vi "Obtain Request Events.vi"(8 "error in":errorcluster, 10 "Create New? (F)":bool) -> (0 "error out":errorcluster, 2 "Core Request Events":T1)   [LabVIEW 2026, in "Core.lvlib"]
doc: "This VI Obtains/Creates the Requests events that will be used for other modules to communicate with the module that owns this VI. These Requests events will be accessed only via Public API methods for this module.\n\n<b>NOTE</b>: The contents of this VI are automatically generated and modified by the <b>Tools > DQMH Consortium > DQMH</b> utilities. Consider using those utilities instead of making your own modifications to this VI.\n_____\nBased on DQMH Dev Tools: Project Template 7.1.2.1547."
uses:
  Core.lvlib
  Request Events--cluster.ctl
  Stop Argument--cluster.ctl
  Show Panel Argument--cluster.ctl
  Hide Panel Argument--cluster.ctl
  Show Diagram Argument--cluster.ctl
  Get Module Execution Status Argument--cluster.ctl
  LaunchEventRecorder Argument--cluster.ctl
  Launcher/Mode.ctl
  Resubscribe to Cloneable Argument--cluster.ctl
  LaunchReplayModule Argument--cluster.ctl
panel:
  # "NOTE: The contents of this VI are automatically generated and modified by the Tools > DQMH Consortium > DQMH utilities. Consider using those utilities instead of making your own modifications to this VI."
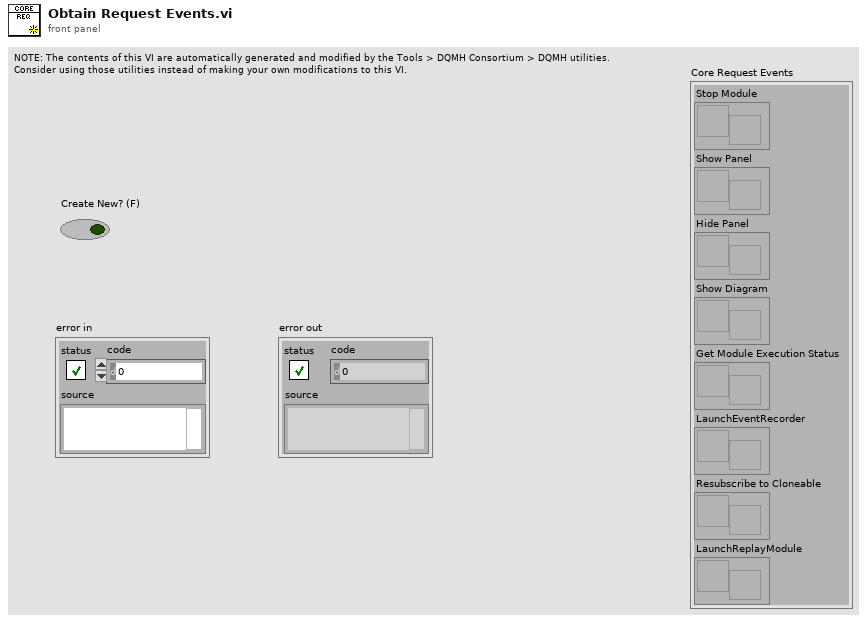
[diagram p1: front panel]
types:
  T1 = typedef "Core.lvlib/Request Events--cluster.ctl" = cluster{"Stop Module":refnum<user-event>, "Show Panel":refnum<user-event>, "Hide Panel":refnum<user-event>, "Show Diagram":refnum<user-event>, "Get Module Execution Status":refnum<user-event>, "LaunchEventRecorder":refnum<user-event>, "Resubscribe to Cloneable":refnum<user-event>, "LaunchReplayModule":refnum<user-event>}
  T2 = typedef "Core.lvlib/LaunchReplayModule Argument--cluster.ctl" = cluster{"Module ID":i32, "Run ID":string}
  T3 = typedef "Core.lvlib/Resubscribe to Cloneable Argument--cluster.ctl" = cluster{"Module ID":i32, "Boolean":bool}
  T4 = typedef "Core.lvlib/LaunchEventRecorder Argument--cluster.ctl" = cluster{"Module ID":i32, "Mode":T5}
  T5 = typedef "Mode.ctl" = enum16{"Record", "Record and Replay"}
  T6 = typedef "Core.lvlib/Get Module Execution Status Argument--cluster.ctl" = cluster{"Module ID":i32, "Running?":bool}
  T7 = typedef "Core.lvlib/Show Diagram Argument--cluster.ctl" = cluster{"Module ID":i32, "Debug?":bool}
  T8 = typedef "Core.lvlib/Show Panel Argument--cluster.ctl" = cluster{"Module ID":i32, "Show Panel?":bool}
  T9 = typedef "Core.lvlib/Hide Panel Argument--cluster.ctl" = cluster{"Module ID":i32, "Hide Panel?":bool}
  T10 = typedef "Core.lvlib/Stop Argument--cluster.ctl" = cluster{"Module ID":i32, "Origin":string, "Exit via Stop Module Req?":bool, "Wait for Module to stop?":bool}
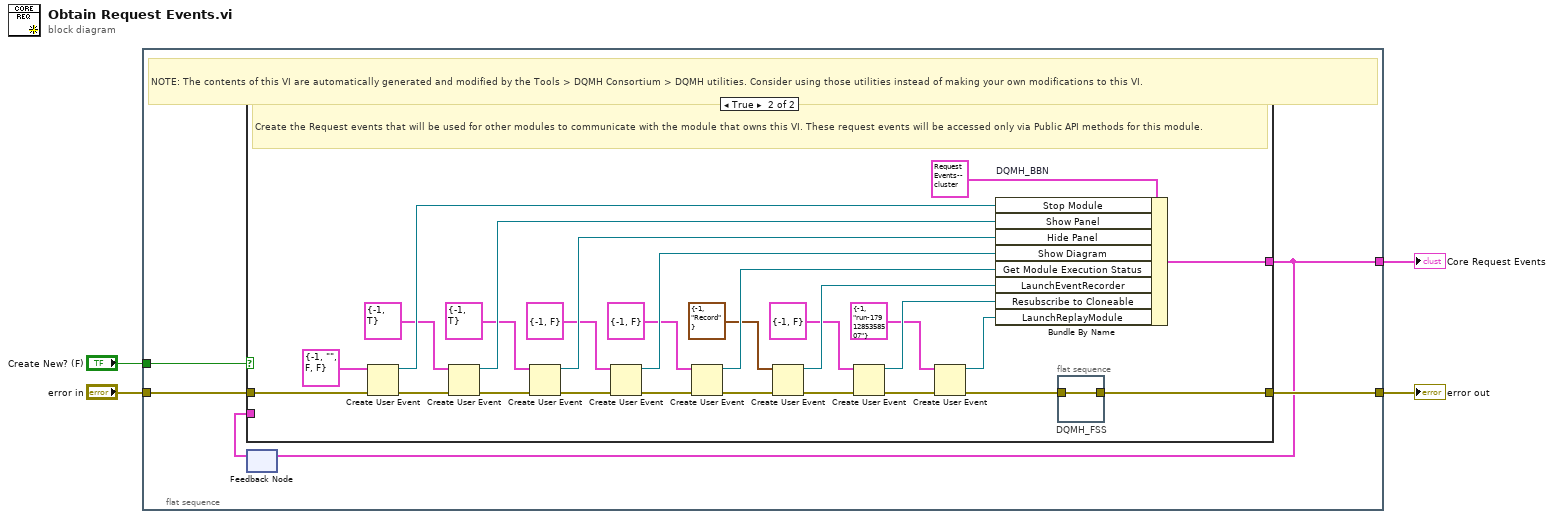
[diagram p0: block diagram]
diagram:
  n1 = flat-sequence {
    tunnel: [w9] -> w4
    tunnel: "error in" -> [w8]
    tunnel: [w6] -> w2
    tunnel: "Create New? (F)" -> [w5]
    frame #0 {
      # "NOTE: The contents of this VI are automatically generated and modified by the Tools > DQMH Consortium > DQMH utilities. Consider using those utilities instead of making your own modifications to this VI."
      n2 = feedback #1() -> (w7:T1)  [unwired: 1 in]
      n3 = case shown="True" w5 {
        tunnel: [w10 w27] -> w9
        tunnel: w8 -> [w10 w39]
        tunnel: [w11 w36] -> w6
        tunnel: w7 -> [w11 _]
        frame False {
        }
        frame True {
          # "Create the Request events that will be used for other modules to communicate with the module that owns this VI. These request events will be accessed only via Public API methods for this module."
          n4 = Create User Event(user event datatype=T10 {"Module ID"=-1, "Origin"="", "Exit via Stop Module Req?"=FALSE, "Wait for Module to stop?"=FALSE} ("Stop Argument"), error in=w39) -> (user event=w37:refnum<user-event>, error out=w34:errorcluster)
          n5 = Create User Event(user event datatype=T8 {"Module ID"=-1, "Show Panel?"=TRUE} ("Show Panel Argument"), error in=w34) -> (user event=w33:refnum<user-event>, error out=w31:errorcluster)
          n6 = Create User Event(user event datatype=T9 {"Module ID"=-1, "Hide Panel?"=TRUE} ("Hide Panel"), error in=w31) -> (user event=w30:refnum<user-event>, error out=w29:errorcluster)
          n7 = Create User Event(user event datatype=T7 {"Module ID"=-1, "Debug?"=FALSE} ("Show Diagram Argument"), error in=w29) -> (user event=w25:refnum<user-event>, error out=w26:errorcluster)
          n8 = Create User Event(user event datatype=T6 {"Module ID"=-1, "Running?"=FALSE} ("Get Module Execution Status Argument"), error in=w26) -> (user event=w22:refnum<user-event>, error out=w23:errorcluster)
          n9 = Create User Event(user event datatype=T4 {"Module ID"=-1, "Mode"=enum."Record"} ("LaunchEventRecorder Argument"), error in=w23) -> (user event=w19:refnum<user-event>, error out=w20:errorcluster)
          n10 = Create User Event(user event datatype=T3 {"Module ID"=-1, "Boolean"=FALSE} ("Resubscribe to Cloneable Argument"), error in=w20) -> (user event=w16:refnum<user-event>, error out=w17:errorcluster)
          n11 = Create User Event(user event datatype=T2 {"Module ID"=-1, "Run ID"="run-1791285358507"} ("LaunchReplayModule Argument"), error in=w17) -> (user event=w13:refnum<user-event>, error out=w14:errorcluster)
          n12 = Bundle By Name "DQMH_BBN"(cluster=T1 {"Stop Module"=refnum, "Show Panel"=refnum, "Hide Panel"=refnum, "Show Diagram"=refnum, "Get Module Execution Status"=refnum, "LaunchEventRecorder"=refnum, "Resubscribe to Cloneable"=refnum, "LaunchReplayModule"=refnum} ("output cluster"), "Stop Module"=w37, "Show Panel"=w33, "Hide Panel"=w30, "Show Diagram"=w25, "Get Module Execution Status"=w22, "LaunchEventRecorder"=w19, "Resubscribe to Cloneable"=w16, "LaunchReplayModule"=w13) -> (w36:T1)
          n13 = flat-sequence "DQMH_FSS" {
            tunnel: w14 -> [w40]
            tunnel: [w40] -> w27
            frame #0 {
            }
          }
        }
      }
      n14 = feedback-in #1(w6) -> ()
    }
  }
  "Core Request Events" <- w2
  "error out" <- w4
